vi "SVXMPL_Force Identical t0.vi"(8 "error in (no error)":errorcluster, 11 "waveforms in":waveform(dbl)[](array[waveform])) -> (0 "error out":errorcluster, 3 "waveforms out":waveform(dbl)[](array[waveform]))   [LabVIEW 2017]
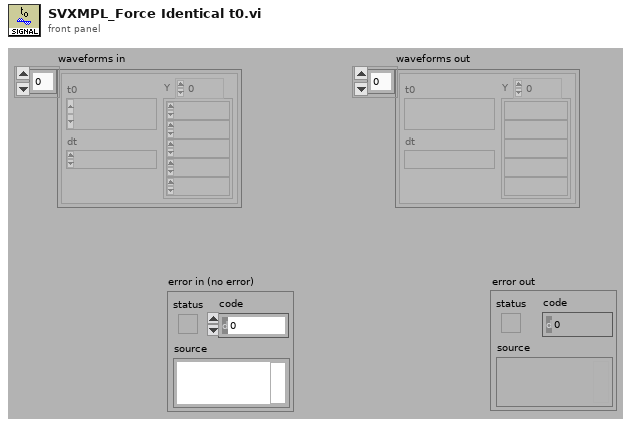
[diagram p1: front panel]
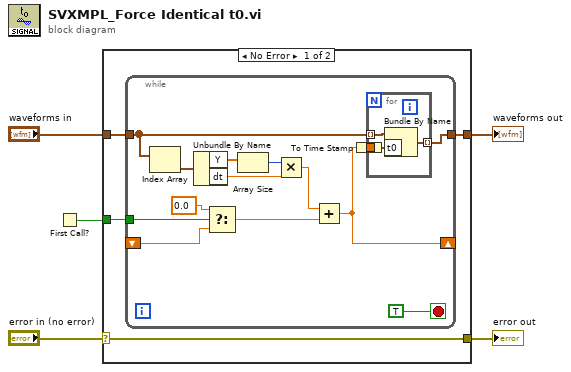
[diagram p0: block diagram]
diagram:
  n1 = First Call?() -> (First Call?: T/F=w1:bool)
  n2 = case shown="No Error" "error in (no error)" {
    selector: "error in (no error)" -> [w9 w28]
    tunnel: [w9 w28] -> w4
    tunnel: "waveforms in" -> [w8 w27]
    tunnel: [w7 w27] -> w2
    tunnel: w1 -> [w6 _]
    frame No Error {
      n3 = while {
        tunnel: w6 -> [w21]
        shift-left: _ -> [w19]
        shift-right: [w10] -> _
        tunnel: [w22] -> w7
        tunnel: w8 -> [w18]
        stop <- TRUE stop-if-true
        n4 = Index Array(array=w18) -> (element=w17:waveform(dbl))  [unwired: 1 in]
        n5 = Unbundle By Name(w17) -> ("Y"=w16:dbl[], "dt"=w14:dbl)
        n6 = Select(t=0.0, s=w21, f=w19) -> (s? t:f=w12:dbl)
        n7 = Array Size(array=w16) -> (size(s)=w15:i32)
        n8 = Multiply(x=w15, y=w14) -> (x*y=w13:dbl)
        n9 = Add(x=w13, y=w12) -> (x+y=w10:dbl)
        n10 = for {
          tunnel: w18 -> [w26] mode=indexing
          tunnel: [w25] -> w22 mode=indexing
          tunnel: w10 -> [w24]
          n11 = To Time Stamp(1:w24) -> (0:w23:timestamp)
          n12 = Bundle By Name(cluster=w26, "t0"=w23) -> (w25:waveform(dbl))
        }
      }
    }
    frame Error {
    }
  }
  "error out" <- w4
  "waveforms out" <- w2
